vi "Read Collected Data1D.vi"(8 "error in (no error)":errorcluster, 11 "AbstractCollector1D in":refnum<class "AbstractCollector1D.lvclass">) -> (0 "error out":errorcluster, 2 "Collected Data":refnum<class "Data1D.lvclass">, 3 "AbstractCollector1D out":refnum<class "AbstractCollector1D.lvclass">)   [LabVIEW 2014, in "AbstractCollector1D.lvclass"]
uses:
  AbstractCollector1D.lvclass
  Model/Data/Data1D/Data1D.lvclass
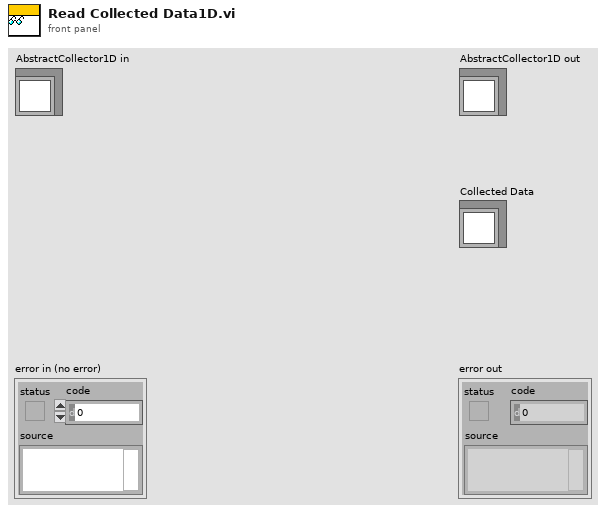
[diagram p1: front panel]
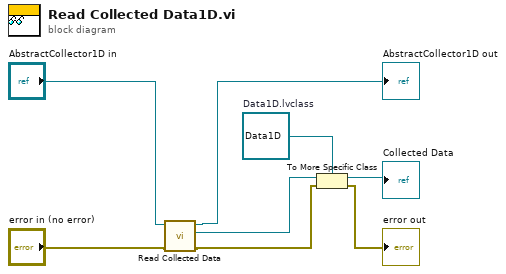
[diagram p0: block diagram]
diagram:
  w7 = refnum<class "Data1D.lvclass"> refnum  # Data1D.lvclass
  n1 = call-dynamic "Read Collected Data.vi"("error in (no error)"="error in (no error)", "AbstractCollector in"="AbstractCollector1D in") -> ("error out"=w3:errorcluster, "Collected Data"=w2:refnum<class "AbstractData.lvclass">, "AbstractCollector out"=→"AbstractCollector1D out":refnum<class "AbstractCollector1D.lvclass">)  [unwired: 7 in]
  n2 = To More Specific Class(target class=w7, reference=w2, error in=w3) -> (specific class reference=→"Collected Data":refnum<class "Data1D.lvclass">, error out=→"error out":errorcluster)
